vi "Read (Waveform)Metodo.vi"(8 "error in (no error)":errorcluster, 9 "Timeout (10000 ms)":u32=10000, 10 "Source (0: Channel 1)":u16(ring) items=["Channel 1", "Channel 2", "Channel 3", "Channel 4", "Math", "Reference A", "Reference B", "Reference C", "Reference D", "FFT"], 11 "Keysight in":refnum<class "Keysight.lvclass">) -> (0 "error out":errorcluster, 2 "Waveform Data":waveform(dbl)(graph), 3 "Keysight out":refnum<class "Keysight.lvclass">)   [LabVIEW 2020, in "Keysight.lvclass"]
uses:
  Keysight.lvclass
  Keysight.lvclass/Keysight.ctl
  <instrlib>/Agilent 2000 3000 X-Series/Agilent 2000 3000 X-Series.lvlib
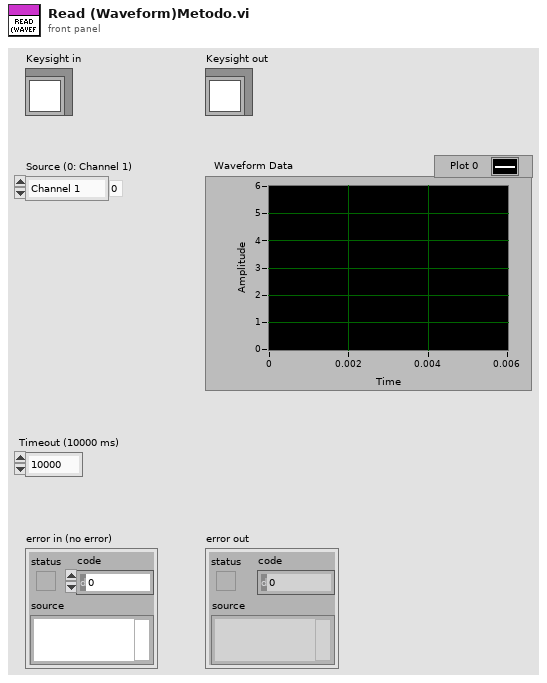
[diagram p1: front panel]
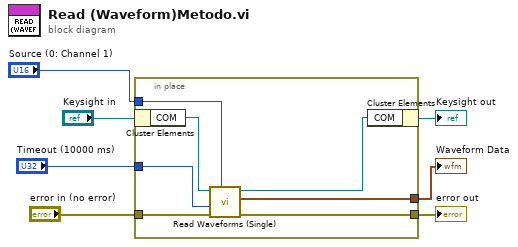
[diagram p0: block diagram]
diagram:
  n1 = in-place {
    in-place-border: [w12] -> w5
    in-place-border: [w11] -> w4
    in-place-border: "error in (no error)" -> [w10]
    in-place-border: "Timeout (10000 ms)" -> [w9]
    in-place-border: "Source (0: Channel 1)" -> [w8]
    n2 = in-place-cluster #1("Keysight in") -> ("COM"=w14:refnum<visa-resource-name>)
    n3 = call <instrlib>:"Read Waveforms (Single).vi"("Bind Source Channel (2: None)"=w8, "error in (no error)"=w10, "Timeout (10000 ms)"=w9, "VISA resource name"=w14) -> ("error out"=w12:errorcluster, "Waveform Data"=w11:waveform(dbl), "VISA resource name out"=w13:refnum<visa-resource-name>)  [unwired: 1 in, 4 out]
    n4 = in-place-cluster #1("COM"=w13) -> (→"Keysight out":refnum<class "Keysight.lvclass">)
  }
  "Waveform Data" <- w4
  "error out" <- w5
